vi "FTW-CodeGen-InitializeCache.vi"(0 "Prototype VI":refnum<vi>, 5 "XRef":refnum<vi>, 11 "error in":errorcluster) -> (6 "Initialized FTW XNode State":T1 {"TotalCodeGens" format="CodeGens:   %04d"; "TotalAdaptToInputs" format="AdaptTerms: %04d"; "FinishedCodegen" format="%_3psec"; "ElapsedTilCodegen" format="%_3psec"; "AdaptToInputsBegin" format="%.3fmsec\n%<%D:%H:%M:%S%3u>t"}, 15 "error out":errorcluster)   [LabVIEW 2015]
uses:
  FTW-CodeGen-XNodeCommonState.ctl
  FTW-CodeGen-XNodeAdaptiveTerminal.ctl
  FTW-CodeGen-XNodeAdaptiveTerminal-Controller.ctl
  src/reflection/FTW-Reflection-Types.ctl
  FTW-CodeGen-XNodeAdaptiveTerminal-ControllerBehavior.ctl
panel:
  # "Inputs"
  # "Outputs"
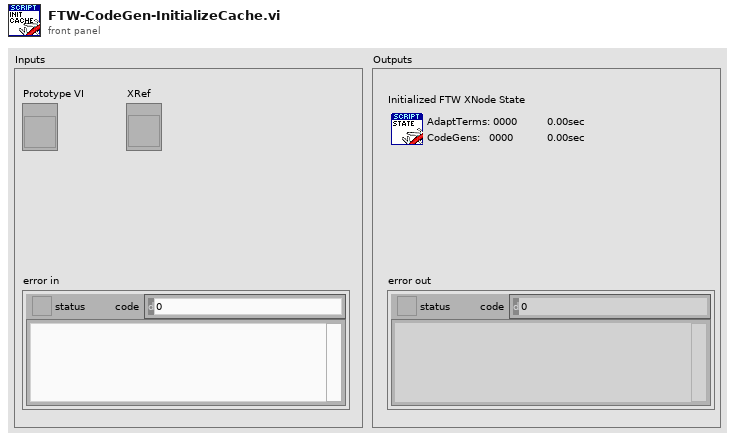
[diagram p1: front panel]
types:
  T1 = typedef "FTW-CodeGen-XNodeCommonState.ctl" = cluster{"Terms":cluster{"Name":string, "Id":string, "Type":variant, "Bounds":cluster{"Left":i32, "Top":i32, "Right":i32, "Bottom":i32}, "Input?":bool, "Required?":bool, "Recommended?":bool, "Adaptive?":bool, "Hidden?":bool, "Direction":enum32{"Auto", "Up", "Down", "Left", "Right", "Center"}, "Break Wire?":bool, "English Name":string}[], "AdaptiveTerms":T2[], "AdaptiveTerminalsOK":bool, "ForceCodeRegeneration?":bool, "LastGeneration":timestamp, "CodeGenError":errorcluster, "AdaptToInputsBegin":dbl, "ElapsedTilCodegen":dbl, "FinishedCodegen":dbl, "TotalAdaptToInputs":i32, "TotalCodeGens":i32}
  T2 = typedef "FTW-CodeGen-XNodeAdaptiveTerminal.ctl" = cluster{"Config":T3, "ID":string, "ParentIndex":i32, "Wired?":bool, "WiredTypeAllowed?":bool, "LastValidWireName":string, "LastValidWireType":T4, "Followers":i32[]}
  T3 = typedef "FTW-CodeGen-XNodeAdaptiveTerminal-Controller.ctl" = cluster{"AllowedTypes":T4[], "UnconstrainedTypeBehavior":T5, "DefaultType":variant}
  T4 = typedef "FTW-Reflection-Types.ctl" = enum16{"Unknown", "Void", "Array", "Cluster", "LVObject", "Boolean", "I8", "I16", "I32", "I64", "U8", "U16", "U32", "U64", "SGL", "DBL", "EXT", "CSG", "CDB", "CXT", "FXP", "EnumU8", "EnumU16", "EnumU32", "EnumU64", "SGLwithUnit", "DBLwithUnit", "EXTwithUnit", "CSGwithUnit", "CDBwithUnit", "CXTwithUnit", "String", "Path", "Picture", "Tag", "LVVariant", "Timestamp", "WaveformI8", "WaveformI16", "WaveformI32", "WaveformI64", "WaveformU8", "WaveformU16", "WaveformU32", "WaveformU64", "WaveformSGL", "WaveformDBL", "WaveformEXT", "WaveformCSG", "WaveformCDB", "WaveformCXT", "WaveformDigital", "WaveformUnknownType", "DigitalData", "DynamicData", "ExternalData", "FileByteStream", "TDMStream", "dotNET", "ActiveX", "VIServerReference", "VIReference", "ApplicationInstance", "Menu", "ConnectionDataSocket", "ConnectionVISA", "ConnectionBluetooth", "ConnectionIrDA", "ConnectionTCP", "ConnectionUDP", "ConnectionHTTPClient", "ConnectionFTP", "Occurrence", "Notifier", "Queue", "Rendezvous", "Semaphore", "RTFIFO", "EventPublisher", "EventRegistration", "EventCallback", "DataValueReference", "GenericClass", "GenericClassTag", "GenericClassDeepCopy", "GenericClassFlattened", "GenericClassTagFlattened", "GenericReferenceType", "WindowsRegistry", "OverloadedDatalogRef", "ReferenceUnknownType", "ByteArray", "ConPaneInterface", "FTWObject"}
  T5 = typedef "FTW-CodeGen-XNodeAdaptiveTerminal-ControllerBehavior.ctl" = enum16{"UseDefaultType", "StickyToLastValidType"}
  T6 = cluster{"Name":string, "Id":string, "Type":variant, "Bounds":cluster{"Left":i32, "Top":i32, "Right":i32, "Bottom":i32}, "Input?":bool, "Required?":bool, "Recommended?":bool, "Adaptive?":bool, "Hidden?":bool, "Direction":enum32{"Auto", "Up", "Down", "Left", "Right", "Center"}, "Break Wire?":bool, "English Name":string}[]
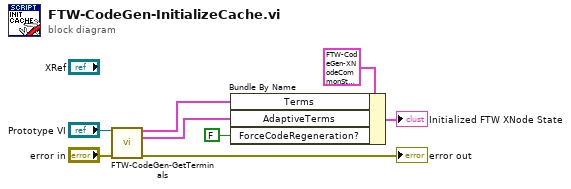
[diagram p0: block diagram]
diagram:
  n1 = call "FTW-CodeGen-GetTerminals.vi"("Prototype VI"="Prototype VI", "error in"="error in") -> ("Terms"=w8:T6, "Adaptive Input Terminals"=w7:T2[], "error out"=→"error out":errorcluster)  [unwired: 11 in]
  n2 = Bundle By Name(cluster=T1 {"Terms"=[], "AdaptiveTerms"=[], "AdaptiveTerminalsOK"=FALSE, "ForceCodeRegeneration?"=FALSE, "LastGeneration"=timestamp(0 s since 1904-01-01), "CodeGenError"={"status"=FALSE, "code"=0, "source"=""}, "AdaptToInputsBegin"=0.0, "ElapsedTilCodegen"=0.0, "FinishedCodegen"=0.0, "TotalAdaptToInputs"=0, "TotalCodeGens"=0} ("Initialized FTW XNode State"), "Terms"=w8, "AdaptiveTerms"=w7, "ForceCodeRegeneration?"=FALSE ("Cache.ForceCodeRegeneration?")) -> (→"Initialized FTW XNode State":T1)
